vi "Script Control To ConPane.vi"(4 "Pane":refnum<vi>, 6 "VI Ref":refnum<vi>, 7 "Terminal Index":i32, 8 "error in":errorcluster, 9 "Wire Rule":T1(ring), 10 "Control To Duplicate":refnum<vi>) -> (0 "error out":errorcluster, 2 "Duplicated Control":refnum<vi>)   [LabVIEW 2025, in "_Rescript.lvlib" / "Msg.lvlib" / "Msg.lvclass"]
uses:
  Msg.lvclass
  Msg.lvclass/Msg.ctl
  _Rescript.lvlib
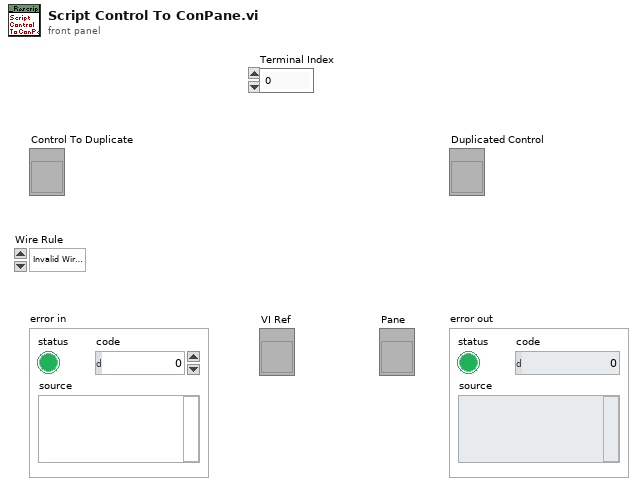
[diagram p1: front panel]
types:
  T1 = enum16{"Invalid Wire Rule", "Required", "Recommended", "Optional", "Dynamic Dispatch"}
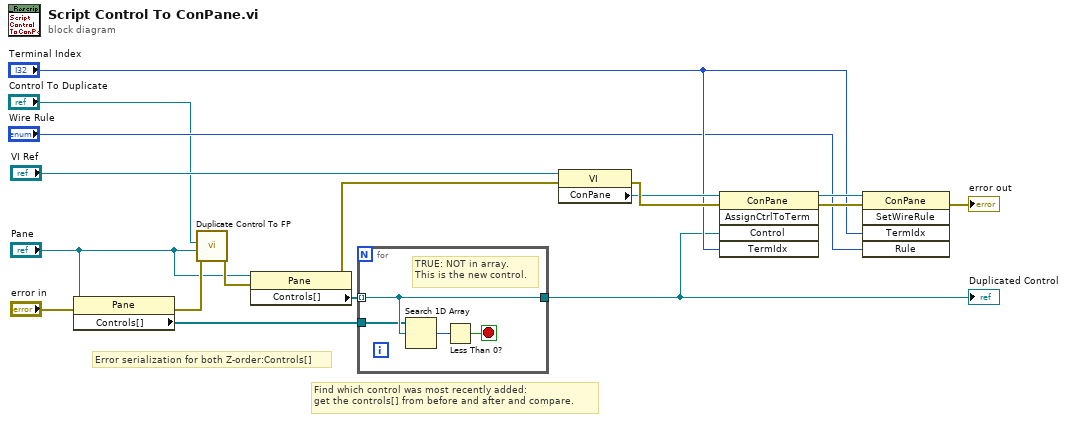
[diagram p0: block diagram]
diagram:
  # "Error serialization for both Z-order:Controls[]"
  # "Find which control was most recently added:\nget the controls[] from before and after and compare."
  n1 = property class="Pane"(reference="Pane", error in="error in") -> (error out=w3:errorcluster, "Controls[]"=w12:refnum<vi>[])  [unwired: 1 out]
  n2 = call "Duplicate Control To FP.vi"("error in"=w3, "Owner"="Pane", "Control"="Control To Duplicate") -> ("error out"=w4:errorcluster)  [unwired: 8 in]
  n3 = property class="Pane"(reference="Pane", error in=w4) -> (error out=w11:errorcluster, "Controls[]"=w13:refnum<vi>[])  [unwired: 1 out]
  n4 = for {
    tunnel: w13 -> [w21] mode=indexing
    tunnel: w12 -> [w20]
    tunnel: [w21] -> w6
    stop <- w18 stop-if-true
    # "TRUE: NOT in array.\nThis is the new control."
    n5 = Search 1D Array(1D array=w20, element=w21) -> (index of element=w19:i32)  [unwired: 1 in]
    n6 = Less Than 0?(x=w19) -> (x < 0?=w18:bool)
  }
  "Duplicated Control" <- w6
  n7 = property class="VI"(reference="VI Ref", error in=w11) -> (error out=w16:errorcluster, "ConPane"=w14:refnum<vi>)  [unwired: 1 out]
  n8 = invoke class="ConPane" method="AssignCtrlToTerm"(reference=w14, error in=w16, "Control"=w6, "TermIdx"="Terminal Index") -> (reference out=w17:refnum<vi>, error out=w15:errorcluster)  [unwired: 1 in, 3 out]
  n9 = invoke class="ConPane" method="SetWireRule"(reference=w17, error in=w15, "TermIdx"="Terminal Index", "Rule"="Wire Rule") -> (error out=→"error out":errorcluster)  [unwired: 1 in, 4 out]
